vi "Read Single Data Point.vi"(8 "error in (no error)":errorcluster, 11 "3446X in":refnum<class "3446X.lvclass">) -> (0 "error out":errorcluster, 2 "Value":dbl, 3 "3446X out":refnum<class "3446X.lvclass">)   [LabVIEW 2018, in "3446X.lvlib" / "3446X.lvclass"]
uses:
  3446X.lvclass
  3446X.lvclass/3446X.ctl
  <instrlib>/Agilent 3446X Series/Public/Data/Read (Single Point).vi
  <instrlib>/Agilent 3446X Series/Agilent 3446X Series.lvlib
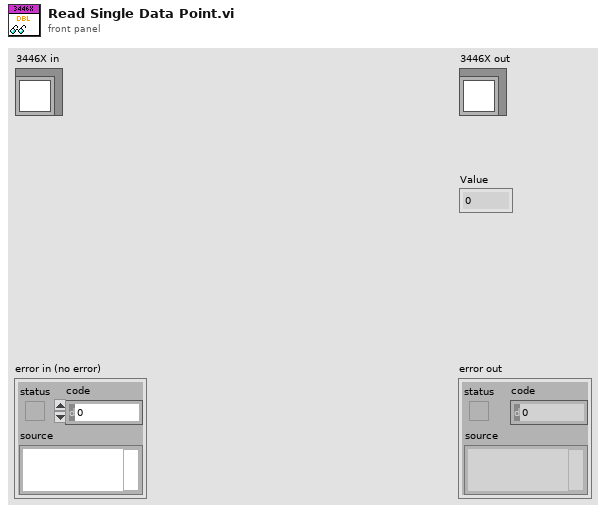
[diagram p1: front panel]
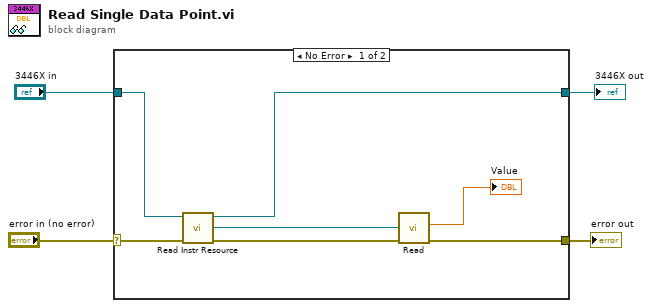
[diagram p0: block diagram]
diagram:
  n1 = case shown="No Error" "error in (no error)" {
    selector: "error in (no error)" -> [w11 w13]
    tunnel: [w6 w13] -> w3
    tunnel: [w9 w12] -> w2
    tunnel: "3446X in" -> [w10 w12]
    frame No Error {
      n2 = call "Read Instr Resource.vi"("error in (no error)"=w11, "3446X in"=w10) -> ("error out"=w7:errorcluster, "Instr Resource"=w8:refnum<visa-resource-name>, "3446X out"=w9:refnum<class "3446X.lvclass">)  [unwired: 7 in]
      n3 = call-poly <instrlib>:"Read.vi"("error in (no error)"=w7, "VISA resource name"=w8) -> ("error out"=w6:errorcluster, "Measurement"=→"Value":dbl)  [unwired: 7 in, 1 out]
    }
    frame Error {
    }
  }
  "error out" <- w3
  "3446X out" <- w2
